vi "Test UNSUBSCRIBE packet.vi"() -> ()   [LabVIEW 2013]
uses:
  source/Control Packets/UNSUBSCRIBE/UNSUBSCRIBE.lvclass
  source/Control Packets/ControlPacket/ControlPacket.lvclass/ControlPacket.ctl
  source/Control Packets/ControlPacket/ControlPacket.lvclass
panel:
  out "Payload":u8[](array[numeric])
  out "Subscription Payload":bool
  out "Packet ID":u16 format="%04x"
  out "error out":errorcluster
  out "Packet Identifier":bool
  out "Packet type":bool
  out "All packets consumed":bool
  out "Complete Packet":bool
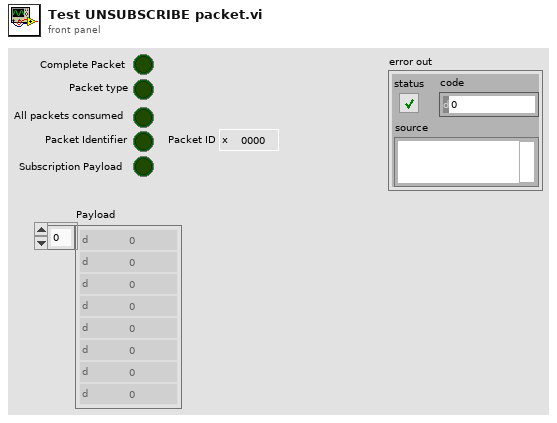
[diagram p1: front panel]
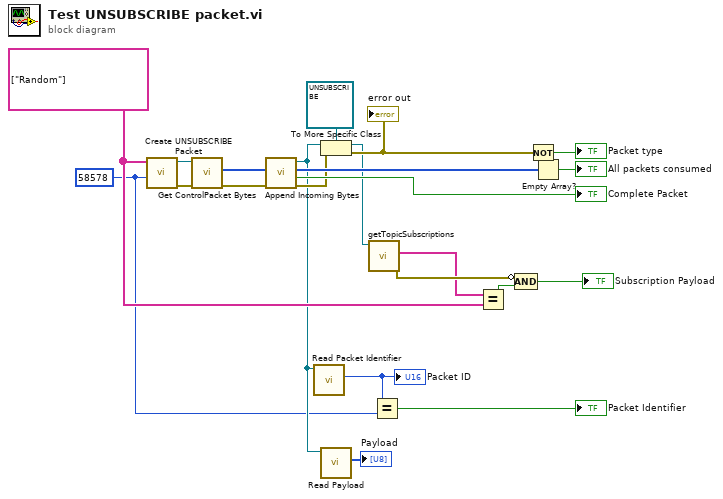
[diagram p0: block diagram]
diagram:
  w7 = string[] ["Random"] ("Topic Subscriptions")
  w1 = u16 58578 ("Packet ID")
  n1 = call "Create UNSUBSCRIBE Packet.vi"("Packet ID (0: generate new)"=w1, "Topic Subscriptions"=w7) -> ("error out"=w9:errorcluster, "UNSUBSCRIBE out"=w8:refnum<class "UNSUBSCRIBE.lvclass">)  [unwired: 8 in]
  n2 = call "Get ControlPacket Bytes.vi"("error in (no error)"=w9, "ControlPacket"=w8) -> ("error out"=w17:errorcluster, "Bytes Stream"=w22:u8[])  [unwired: 7 in, 1 out]
  n3 = call "Append Incoming Bytes.vi"("error in (no error)"=w17, "Incoming Packets"=w22) -> ("error out"=w16:errorcluster, "Complete Packet"=→"Complete Packet":bool, "Remaining Packets"=w20:u8[], "ControlPacket"=w3:refnum<class "ControlPacket.lvclass">)  [unwired: 6 in]
  n4 = call "Read Packet Identifier.vi"("ControlPacket in"=w3) -> ("Packet Identifier"=w15:u16)  [unwired: 9 in, 1 out]
  "Packet ID" <- w15
  n5 = To More Specific Class(target class=refnum<class "UNSUBSCRIBE.lvclass"> refnum ("UNSUBSCRIBE.lvclass"), reference=w3, error in=w16) -> (specific class reference=w6:refnum<class "UNSUBSCRIBE.lvclass">, error out=w13:errorcluster)
  "error out" <- w13
  n6 = call "Read Payload.vi"("ControlPacket in"=w3) -> ("Payload"=→"Payload":u8[])  [unwired: 9 in, 1 out]
  n7 = call "getTopicSubscriptions.vi"("UNSUBSCRIBE in"=w6) -> ("error out"=w5:errorcluster, "Topic Subscriptions"=w4:string[])  [unwired: 8 in, 1 out]
  n8 = Equal?(x=w15, y=w1) -> (x = y?=→"Packet Identifier":bool)
  n9 = Equal?(x=w4, y=w7) -> (x = y?=w12:bool)
  n10 = Compound Arithmetic op=AND(invert w5, w12) -> (→"Subscription Payload":bool)
  n11 = Not(x=w13) -> (.not. x?=→"Packet type":bool)
  n12 = Empty Array?(array=w20) -> (empty?=→"All packets consumed":bool)
